vi "testWaitTimerWithCheckWaitRate.vi"(8 "error in (no error)":errorcluster, 11 "testStateMachineUtilities in":refnum<class "testStateMachineUtilities.lvclass">) -> (0 "error out":errorcluster, 3 "testStateMachineUtilities out":refnum<class "testStateMachineUtilities.lvclass">)   [LabVIEW 2013, in "testStateMachineUtilities.lvclass"]
uses:
  testStateMachineUtilities.lvclass
  <vilib>/Utility/error.llb/Error Cluster From Error Code.vi
panel:
  out "Array":string[](array[string])
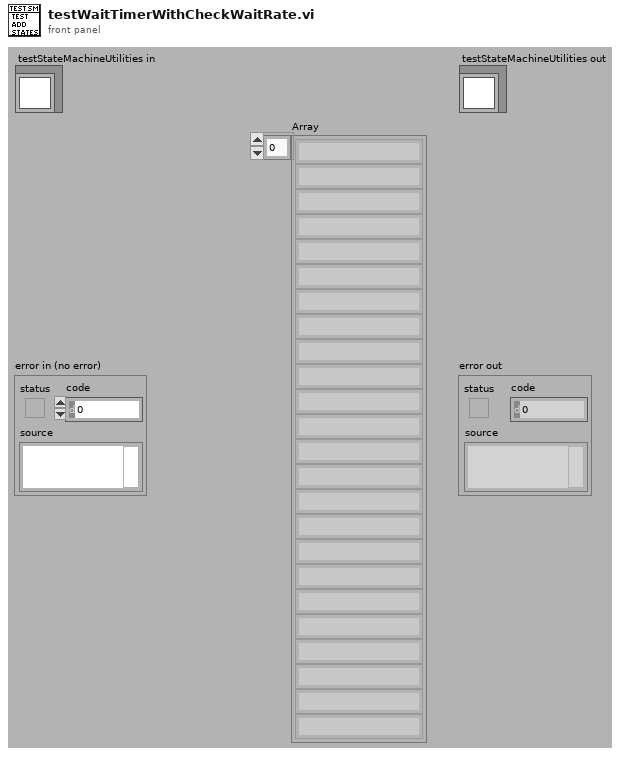
[diagram p1: front panel]
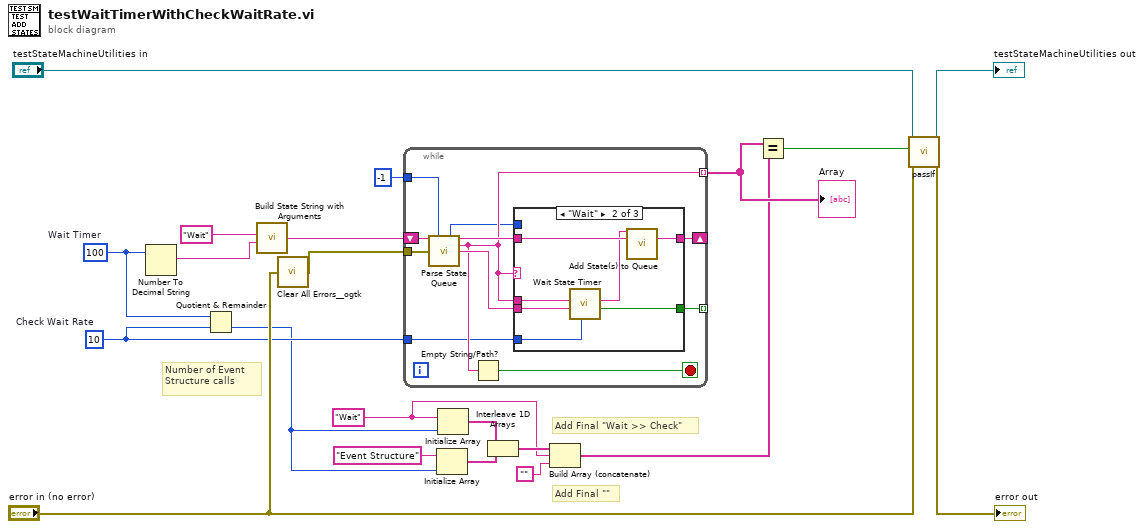
[diagram p0: block diagram]
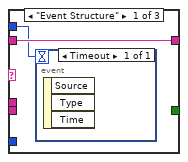
[diagram p2: hidden frame]
diagram:
  w11 = 100  # Wait Timer
  w10 = 10  # Check Wait Rate
  w4 = "Wait" ("State Queue")
  # "Number of Event Structure calls"
  # "Add Final \"\""
  # "Add Final \"Wait >> Check\""
  n1 = Number To Decimal String(number=w11) -> (decimal integer string=w13:string)  [unwired: 1 in]
  n2 = Quotient & Remainder(x=w11, y=w10) -> (floor(x/y)=w8:i32)  [unwired: 1 out]
  n3 = call "Build State String with Arguments.vi"("Arguments (\"\")"=w13, "State"="Wait" ("State Queue")) -> ("State with Arguments"=w12:string)  [unwired: 4 in]
  n4 = call <userlib>:"Clear All Errors__ogtk.vi"("Error In"="error in (no error)") -> ("Error Out"=w17:errorcluster)  [unwired: 3 in]
  n5 = while {
    tunnel: w17 -> [w31]
    shift-right: [w25] -> _
    shift-left: w12 -> [w32]
    tunnel: -1 ("Timeout") -> [w30]
    tunnel: [w24] -> w2 mode=indexing
    tunnel: [w27] -> _ mode=indexing
    tunnel: w10 -> [w22]
    stop <- w29 stop-if-true
    n6 = call "Parse State Queue.vi"("State Queue"=w32, "Timeout"=w30, "Error In (no error)"=w31) -> ("Timeout out"=w23:i32, "Remaining States"=w26:string, "Current State"=w24:string, "Arguments"=w28:string)  [unwired: 9 in]
    n7 = Empty String/Path?(string/path=w24) -> (empty?=w29:bool)
    n8 = case shown="\"Wait\"" w24 {
      tunnel: w24 -> [_ w41 _]
      tunnel: w28 -> [_ w40 _]
      tunnel: [_ w39 _] -> w27
      tunnel: w26 -> [w34 w38 w42]
      tunnel: [w34 w37 w42] -> w25
      tunnel: w22 -> [_ w35 _]
      tunnel: w23 -> [w33 _ _]
      frame "Event Structure" {
        n9 = event shown="[0] Timeout" {
          selector: _ -> [_]
          dyn-events: _ -> [_]
          timeout: w33 -> [_]
          event Timeout {
            n10 = event-data() -> ()  [unwired: 1 in, 3 out]
          }
        }
      }
      frame "Wait" {
        n11 = call "Wait State Timer.vi"("Check Wait Rate"=w35, "Wait Time (Decimal String)"=w40, "Current State"=w41) -> ("Wait Timer Elapsed"=w39:bool, "States to Enqueue"=w36:string)  [unwired: 5 in, 2 out]
        n12 = call "Add State(s) to Queue.vi"("State(s) in Front (\"\")"=w36, "State(s) in (\"\")"=w38) -> ("States Out"=w37:string)  [unwired: 13 in]
      }
      frame Default {
      }
    }
  }
  "Array" <- w2
  n13 = Initialize Array("Event Structure" ("State Queue"), w8) -> (w6:string[])
  n14 = Initialize Array(w4, w8) -> (w7:string[])
  n15 = Interleave 1D Arrays(w7, w6) -> (w5:string[])
  n16 = Build Array (concatenate)(w5, w4, "") -> (w1:string[])
  n17 = Equal?(x=w2, y=w1) -> (x = y?=w15:bool)
  n18 = call-dynamic "passIf.vi"("error in (no error)"="error in (no error)", "pass"=w15, "TestCase in"="testStateMachineUtilities in") -> ("error out"=→"error out":errorcluster, "TestCase out"=→"testStateMachineUtilities out":refnum<class "testStateMachineUtilities.lvclass">)  [unwired: 7 in]
